vi "FGV Serial.vi"(7 "VISA resource name":refnum<visa-resource-name>="COM3", 8 "error in (no error)":errorcluster, 10 "String":string="H", 11 "Task":T1) -> (0 "error out":errorcluster, 1 "Text output":i32, 3 "return count":u32)   [LabVIEW 2014]
uses:
  control/FGV Serial Tasks.ctl
  <vilib>/Instr/_visa.llb/VISA Flush IO Buffer Mask.ctl
  <vilib>/Instr/_visa.llb/VISA Configure Serial Port (Instr).vi
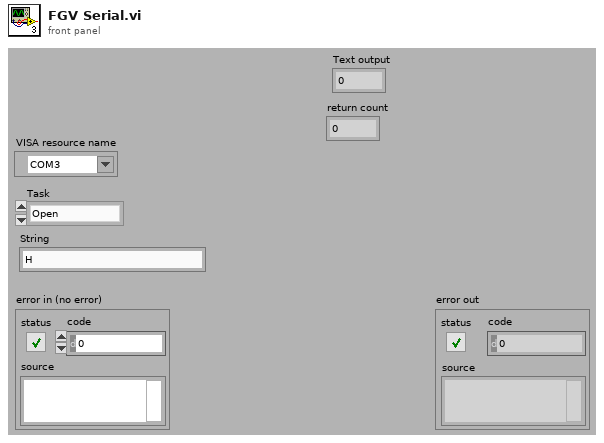
[diagram p1: front panel]
types:
  T1 = typedef "FGV Serial Tasks.ctl" = enum16{"Open", "Read", "Write", "Close", "Flush"}
  T2 = typedef "VISA Flush IO Buffer Mask.ctl" = u16
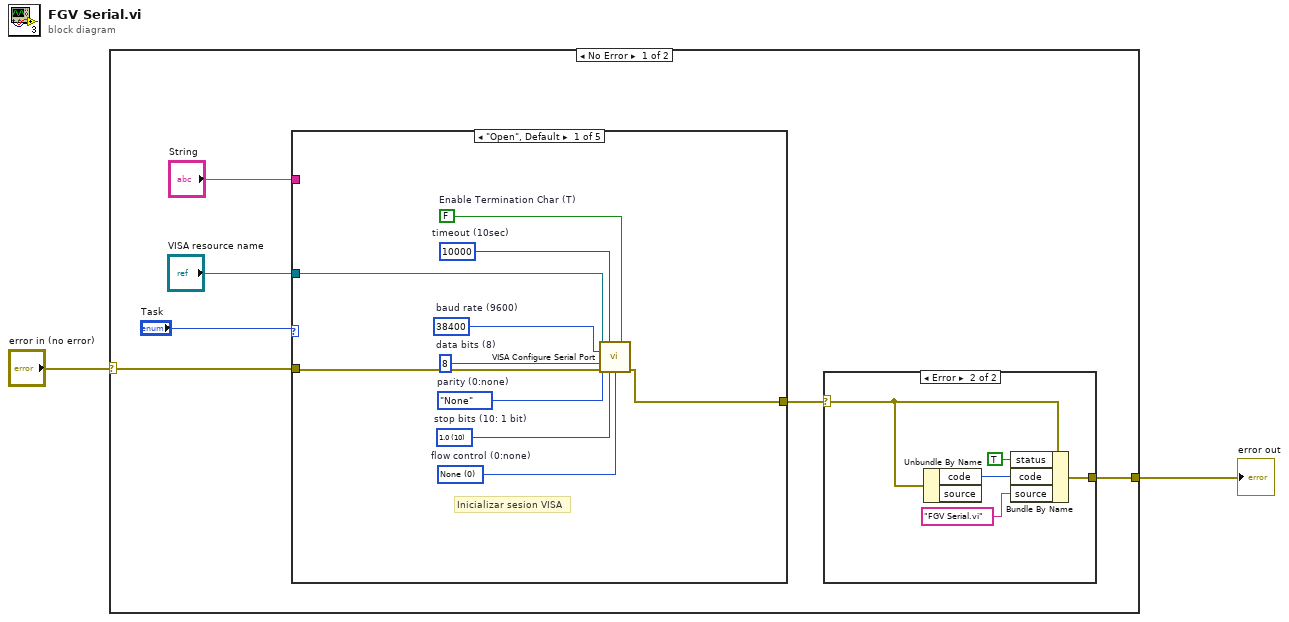
[diagram p0: block diagram]
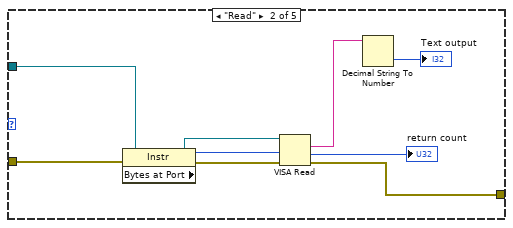
[diagram p3: hidden frame]
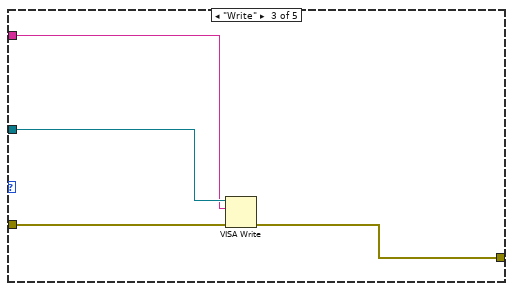
[diagram p4: hidden frame]
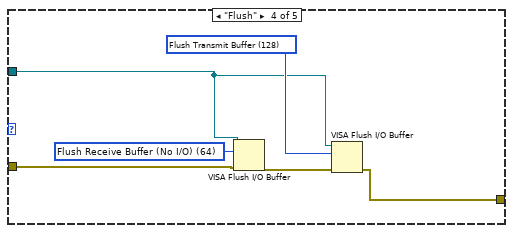
[diagram p5: hidden frame]
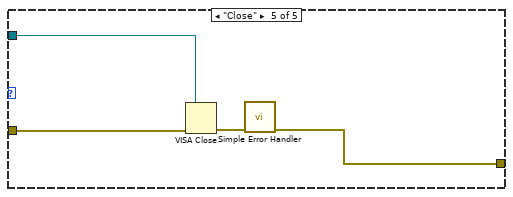
[diagram p6: hidden frame]
diagram:
  n1 = case shown="No Error" "error in (no error)" {
    selector: "error in (no error)" -> [w7 w48]
    tunnel: [w3 w48] -> w1
    frame No Error {
      n2 = case shown="\"Open\", Default" "Task" {
        tunnel: "VISA resource name" -> [w17 w33 w35 w40 w44]
        tunnel: [w16 w28 w36 w38 w45] -> w4
        tunnel: w7 -> [w15 w32 w37 w43 w46]
        tunnel: "String" -> [_ _ w34 _ _]
        frame "Open", Default {
          w22 = u16 0 items=["None", "XON/XOFF", "RTS/CTS", "XON/XOFF & RTS/CTS", "DTR/DSR", "XON/XOFF & DTR/DSR"]  # flow control (0:none)
          w21 = u16 10 items=["1.0"=10, "1.5"=15, "2.0"=20]  # stop bits (10: 1 bit)
          w20 = enum16{"None", "Odd", "Even", "Mark", "Space"}."None"  # parity (0:none)
          w19 = u16 8  # data bits (8)
          w18 = u32 38400  # baud rate (9600)
          w23 = u32 10000  # timeout (10sec)
          w24 = FALSE  # Enable Termination Char (T)
          # "Inicializar sesion VISA"
          n3 = call-poly "VISA Configure Serial Port"("VISA resource name"=w17, "timeout (10sec)"=w23, "Enable Termination\nChar (T)"=w24, "baud rate (9600)"=w18, "data bits (8)"=w19, "parity (0:none)"=w20, "error in (no error)"=w15, "stop bits (10: 1 bit)"=w21, "flow control (0:none)"=w22) -> ("error out"=w16:errorcluster)  [unwired: 5 in, 1 out]
        }
        frame "Read" {
          n4 = property class="Instr"(reference=w33, error in=w32) -> (reference out=w31:refnum<visa-resource-name>, error out=w29:errorcluster, "Bytes at Port"=w30:u32)
          n5 = VISA Read(VISA resource name=w31, byte count=w30, error in (no error)=w29) -> (read buffer=w26:string, return count=→"return count":u32, error out=w28:errorcluster)  [unwired: 1 out]
          n6 = Decimal String To Number(string=w26) -> (number=→"Text output":i32)  [unwired: 2 in, 1 out]
        }
        frame "Write" {
          n7 = VISA Write(VISA resource name=w35, write buffer=w34, error in (no error)=w37) -> (error out=w36:errorcluster)  [unwired: 2 out]
        }
        frame "Flush" {
          w41 = T2 128 items=["Flush Receive Buffer"=16, "Write Transmit Buffer to Device"=32, "Flush Receive Buffer (No I/O)"=64, "Flush Transmit Buffer"=128] ("Mask")
          w42 = T2 64 items=["Flush Receive Buffer"=16, "Write Transmit Buffer to Device"=32, "Flush Receive Buffer (No I/O)"=64, "Flush Transmit Buffer"=128] ("Mask")
          n8 = VISA Flush I/O Buffer(VISA resource name=w40, mask (16)=w42, error in (no error)=w43) -> (error out=w39:errorcluster)  [unwired: 1 out]
          n9 = VISA Flush I/O Buffer(VISA resource name=w40, mask (16)=w41, error in (no error)=w39) -> (error out=w38:errorcluster)  [unwired: 1 out]
        }
        frame "Close" {
          n10 = VISA Close(VISA resource name=w44, error in (no error)=w46) -> (error out=w47:errorcluster)
          n11 = call <vilib>:"Simple Error Handler.vi"("error in (no error)"=w47) -> ("error out"=w45:errorcluster)  [unwired: 4 in, 4 out]
        }
      }
      n12 = case shown="Error" w4 {
        selector: w4 -> [w9 w13]
        tunnel: [w9 w12] -> w3
        frame No Error {
        }
        frame Error {
          n13 = Unbundle By Name(w13) -> ("code"=w14:i32)  [unwired: 1 out]
          n14 = Bundle By Name(cluster=w13, "status"=TRUE, "code"=w14, "source"="FGV Serial.vi") -> (w12:errorcluster)
        }
      }
    }
    frame Error {
    }
  }
  "error out" <- w1
